vi "GetAllGlinks.vi"(2 "sdf in":string, 3 "Model In":refnum<vi>) -> (0 "remaining":string, 1 "Model Out":refnum<vi>)   [LabVIEW 2010]
uses:
  <vilib>/picture/3D Picture Control/NI_3D Picture Control.lvlib
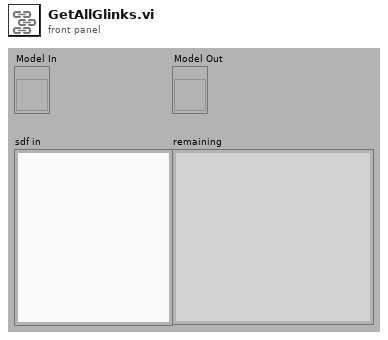
[diagram p1: front panel]
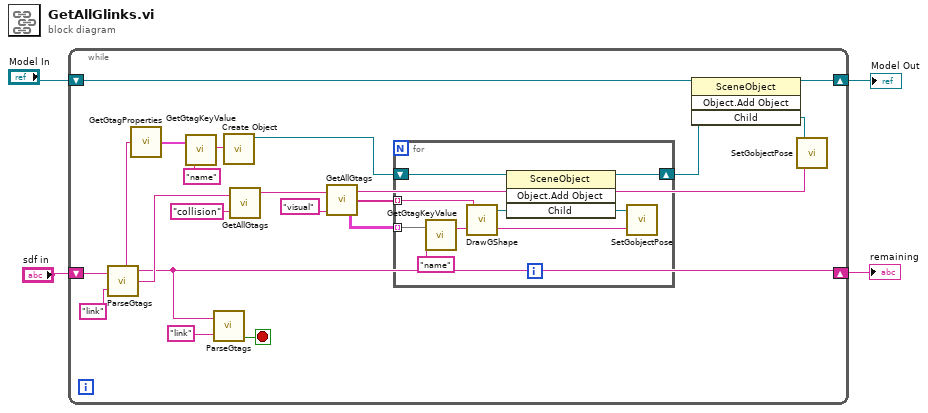
[diagram p0: block diagram]
diagram:
  n1 = while {
    shift-right: [w11] -> w2
    shift-left: "sdf in" -> [w25]
    shift-right: [w7] -> w4
    shift-left: "Model In" -> [w8]
    stop <- w9 stop-if-true
    n2 = call "ParseGtags.vi"("tag"="link", "urdf in"=w25) -> ("parameters"=w23:string, "contents"=w22:string, "urdf out"=w11:string)  [unwired: 1 out]
    n3 = call "GetGtagProperties.vi"("parameters"=w23) -> ("Parameters"=w20:cluster{"key":string, "value":string}[])
    n4 = call "GetGtagKeyValue.vi"("tag"="name", "parameters"=w20) -> ("value"=w13:string)
    n5 = call "ParseGtags.vi"("tag"="link", "urdf in"=w11) -> ("not found"=w9:bool)  [unwired: 3 out]
    n6 = call <vilib>:"Create Object.vi"("Name"=w13) -> ("Scene:New Object"=w12:refnum<vi>)  [unwired: 1 in, 9 out]
    n7 = call "GetAllGtags.vi"("tag"="collision", "sdf in"=w22) -> ("sdf left"=w18:string)  [unwired: 2 out]
    n8 = call "GetAllGtags.vi"("tag"="visual", "sdf in"=w18) -> ("Parameters"=w15:cluster{"key":string, "value":string}[][], "contents"=w16:string[], "sdf left"=w14:string)
    n9 = for {
      tunnel: w16 -> [w31] mode=indexing
      shift-right: [w28] -> w6
      shift-left: w12 -> [w29]
      tunnel: w15 -> [w33] mode=indexing
      n10 = call "GetGtagKeyValue.vi"("tag"="name", "parameters"=w33) -> ("value"=w32:string)
      n11 = call "DrawGShape.vi"("name"=w32, "contents"=w31) -> ("remaining"=w30:string, "Object out"=w27:refnum<vi>)
      n12 = invoke class="SceneObject" method="Object.Add Object"(reference=w29, "Child"=w27) -> (reference out=w28:refnum<vi>, "Child"=w26:refnum<vi>)  [unwired: 2 in, 2 out]
      n13 = call "SetGobjectPose.vi"("contents"=w30, "Object in"=w26) -> ()  [unwired: 2 out]
    }
    n14 = invoke class="SceneObject" method="Object.Add Object"(reference=w8, "Child"=w6) -> (reference out=w7:refnum<vi>, "Child"=w5:refnum<vi>)  [unwired: 2 in, 2 out]
    n15 = call "SetGobjectPose.vi"("contents"=w14, "Object in"=w5) -> ()  [unwired: 2 out]
  }
  "Model Out" <- w4
  "remaining" <- w2
